vi "Save Method VIs.vi"(10 "Class Methods":refnum<vi>[](array[refnum]), 11 "LVClass":refnum<vi>) -> (3 "LVClass Dup":refnum<vi>)   [LabVIEW 2013]
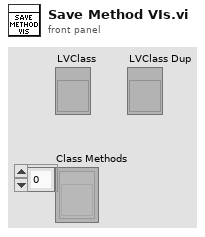
[diagram p1: front panel]
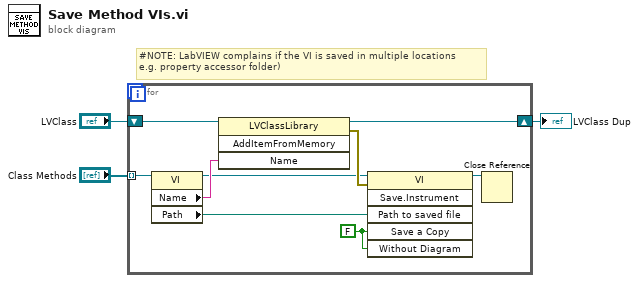
[diagram p0: block diagram]
diagram:
  # "#NOTE: LabVIEW complains if the VI is saved in multiple locations\ne.g. property accessor folder)"
  n1 = for {
    tunnel: "Class Methods" -> [w11] mode=indexing
    shift-right: [w9] -> w2
    shift-left: "LVClass" -> [w10]
    w12 = FALSE ("Save a Copy")
    # "Save VIs that aren't property accessors"
    n2 = property class="VI"(reference=w11) -> (reference out=w4:refnum<vi>, "Name"=w6:string, "Path"=w5:path)  [unwired: 1 in, 1 out]
    n3 = invoke class="LVClassLibrary" method="AddItemFromMemory"(reference=w10, "Name"=w6) -> (reference out=w9:refnum<vi>, error out=w8:errorcluster)  [unwired: 2 in, 2 out]
    n4 = invoke class="VI" method="Save.Instrument"(reference=w4, error in=w8, "Path to saved file"=w5, "Save a Copy"=w12, "Without Diagram"=w12) -> (reference out=w7:refnum<vi>)  [unwired: 1 in, 5 out]
    n5 = Close Reference(reference=w7) -> ()  [unwired: 1 in, 1 out]
  }
  "LVClass Dup" <- w2
